vi "RedefineMasterIP.vi"() -> (1 "Abort?":bool, 2 "Start Master":bool)   [LabVIEW 2012]
doc: "Returns the current Master IP and port.\n\nUser has the option to change the address and/or port or make themselves the master"
uses:
  <userlib>/ROSforLV/ROS/Code/_ROSDefinition.vi
panel:
  in  "Master":bool
  in  "Cancel Button":bool
  in  "OK Button":bool
  in  "Address":string(combo)
  # "Please enter your Master IP address."
  # "Make me Master"
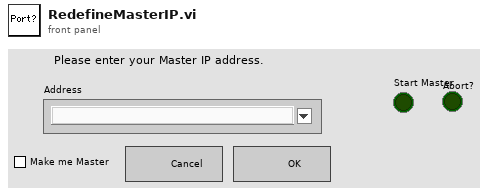
[diagram p1: front panel]
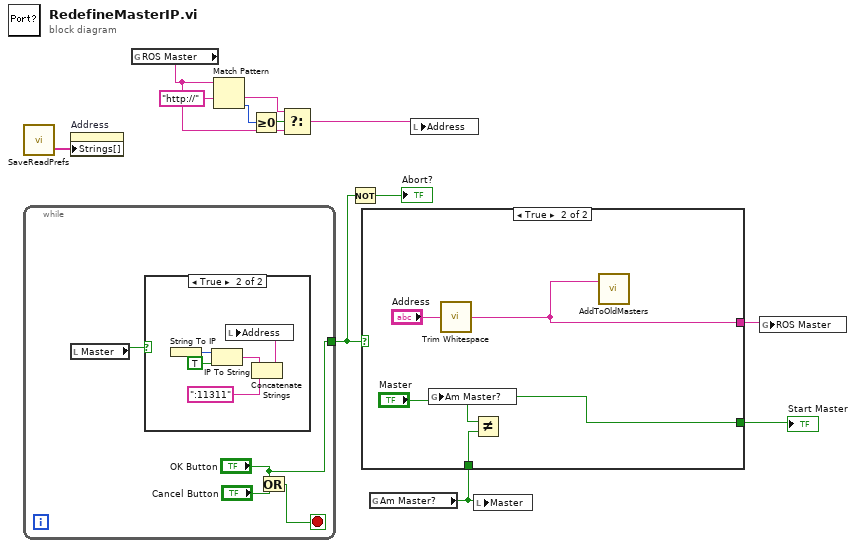
[diagram p0: block diagram]
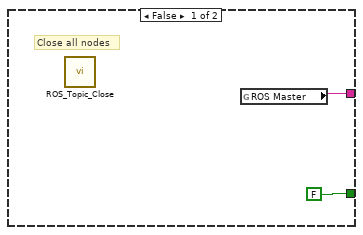
[diagram p3: hidden frame]
diagram:
  n1 = call <userlib>:"SaveReadPrefs.vi"() -> ("Masters"=w2:string[])  [unwired: 3 in]
  n2 = while {
    tunnel: ["OK Button"] -> w12
    stop <- w15 stop-if-true
    n3 = local read "Master"() -> (w13:bool)
    n4 = case shown="True" w13 {
      frame False {
      }
      frame True {
        n5 = String To IP() -> (0:w21:u32)  [unwired: 1 in]
        n6 = IP To String(1:TRUE ("dot notation? (F)"), 2:w21) -> (0:w19:string)
        n7 = Concatenate Strings(w19, ":11311" ("Port")) -> (w17:string)
        n8 = local write "Address"(w17) -> ()
      }
    }
    n9 = Or(x="OK Button", y="Cancel Button") -> (x .or. y?=w15:bool)
  }
  n10 = property on="Address" class="CmbBox"("Strings[]"=w2) -> ()  [unwired: 2 in, 2 out]
  n11 = global read "_ROSDefinition.vi" "ROS Master"() -> (w3:string)
  n12 = Match Pattern(string=w3, regular expression="http://") -> (after substring=w4:string, offset past match=w6:i32)  [unwired: 1 in, 2 out]
  n13 = Greater Or Equal To 0?(x=w6) -> (x >= 0?=w5:bool)
  n14 = Select(t=w4, s=w5, f=w3) -> (s? t:f=w1:string)
  n15 = Not(x=w12) -> (.not. x?=→"Abort?":bool)
  n16 = global read "_ROSDefinition.vi" "Am Master?"() -> (w9:bool)
  n17 = case shown="True" w12 {
    tunnel: [w23 w24] -> w11
    tunnel: w9 -> [_ w27]
    tunnel: [FALSE "Master"] -> w8
    frame False {
      # "Close all nodes"
      n18 = call <userlib>:"ROS_Topic_Close.vi"() -> ()  [unwired: 4 in, 1 out]
      n19 = global read "_ROSDefinition.vi" "ROS Master"() -> (w23:string)
    }
    frame True {
      n20 = global write "_ROSDefinition.vi" "Am Master?"("Master") -> ()
      n21 = call <vilib>:"Trim Whitespace.vi"("string"="Address") -> ("trimmed string"=w24:string)  [unwired: 1 in]
      n22 = Not Equal?(x="Master", y=w27) -> ()  [unwired: 1 out]
      n23 = call <userlib>:"AddToOldMasters.vi"("Address"=w24) -> ()  [unwired: 3 in]
    }
  }
  "Start Master" <- w8
  n24 = local write "Address"(w1) -> ()
  n25 = local write "Master"(w9) -> ()
  n26 = global write "_ROSDefinition.vi" "ROS Master"(w11) -> ()
